vi "Entry_QueueOperations_FGV.vi"(8 "error in":errorcluster, 10 "Data":T1, 11 "Action":T3) -> (0 "error out":errorcluster, 1 "#elements in queue":i32, 2 "elements in queue":T1[](array[typedef]), 3 "queue ref":refnum<queue>)   [LabVIEW 2019]
uses:
  #typedef_Queue_enum.ctl
  #typedef_Data_Entry.ctl
  #typedef_EntryConsole_Action_enum.ctl
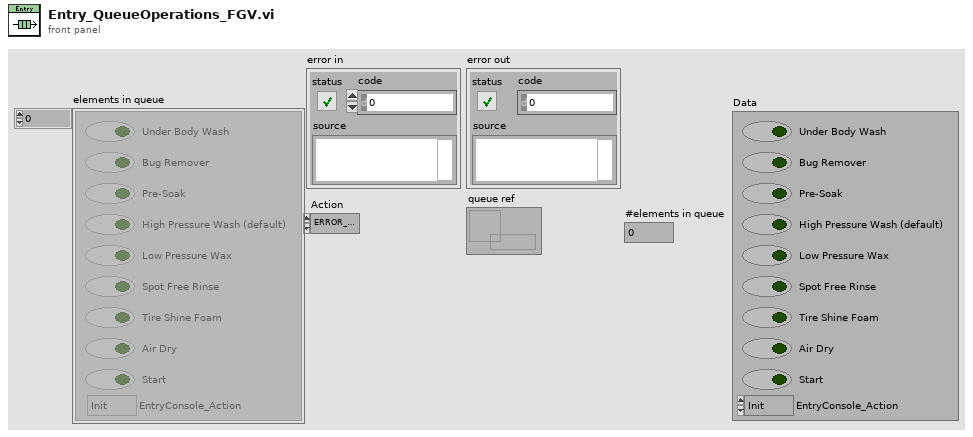
[diagram p1: front panel]
types:
  T1 = typedef "#typedef_Data_Entry.ctl" = cluster{"Under Body Wash":bool, "Bug Remover":bool, "Pre-Soak":bool, "High Pressure Wash (default)":bool, "Low Pressure Wax":bool, "Spot Free Rinse":bool, "Tire Shine Foam":bool, "Air Dry":bool, "Start":bool, "EntryConsole_Action":T2}
  T2 = typedef "#typedef_EntryConsole_Action_enum.ctl" = enum16{"Init", "ERROR_DEFAULT", "Idle", "Pending_Wash_Cycle", "Clear_Console", "Close", "Error_Handler", "Exit"}
  T3 = typedef "#typedef_Queue_enum.ctl" = enum16{"ERROR_default", "Obtain", "Enqueue", "GetStatus", "Flush", "Release"}
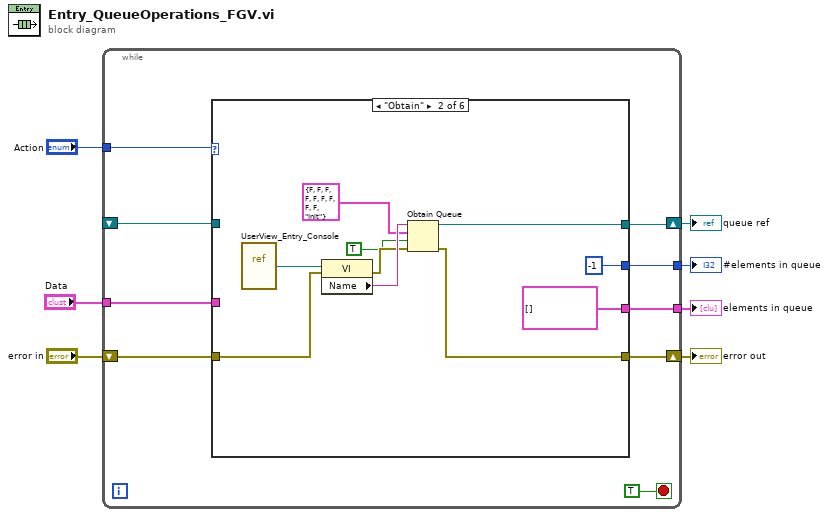
[diagram p0: block diagram]
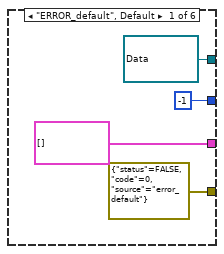
[diagram p2: hidden frame]
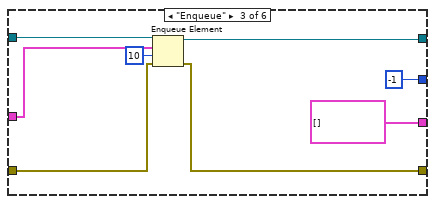
[diagram p3: hidden frame]
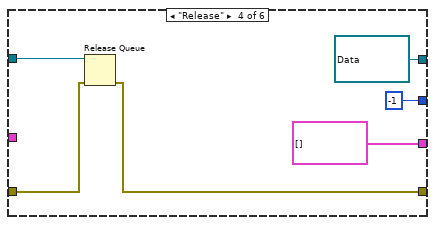
[diagram p4: hidden frame]
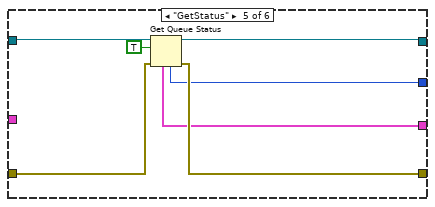
[diagram p5: hidden frame]
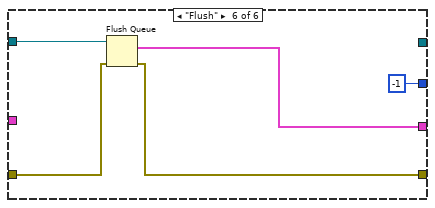
[diagram p6: hidden frame]
diagram:
  n1 = while {
    tunnel: "Action" -> [w15]
    tunnel: "Data" -> [w13]
    tunnel: [w10] -> w1
    shift-right: [w11] -> w3
    shift-left: _ -> [w9]
    shift-right: [w12] -> w5
    shift-left: "error in" -> [w14]
    tunnel: [w8] -> w2
    stop <- TRUE stop-if-true
    n2 = case shown="\"Obtain\"" w15 {
      tunnel: w14 -> [_ w30 w37 w43 w48 w55]
      tunnel: w13 -> [_ _ w33 _ _ _]
      tunnel: [errorcluster {"status"=FALSE, "code"=0, "source"="error_default"} ("error out") w27 w36 w42 w49 w54] -> w12
      tunnel: [refnum<queue> refnum ("queue out") w22 w35 refnum<queue> refnum ("queue out") w50 _] -> w11
      tunnel: [-1 ("# elements in queue") -1 ("#elements in queue") -1 ("#elements in queue") -1 ("# elements in queue") w47 -1 ("# elements in queue")] -> w10
      tunnel: w9 -> [_ _ w38 w44 w51 w56]
      tunnel: [T1[] [] ("Array") T1[] [] ("Array") T1[] [] ("Array") T1[] [] ("Array") w46 w52] -> w8
      frame "ERROR_default", Default {
      }
      frame "Obtain" {
        n3 = vi-ref "UserView_Entry_Console.vi"() -> (w24:refnum<vi>)
        n4 = property class="VI"(reference=w24, error in=w30) -> (error out=w28:errorcluster, "Name"=w29:string)  [unwired: 1 out]
        n5 = Obtain Queue(name (unnamed)=w29, element data type=T1 {"Under Body Wash"=FALSE, "Bug Remover"=FALSE, "Pre-Soak"=FALSE, "High Pressure Wash (default)"=FALSE, "Low Pressure Wax"=FALSE, "Spot Free Rinse"=FALSE, "Tire Shine Foam"=FALSE, "Air Dry"=FALSE, "Start"=FALSE, "EntryConsole_Action"=enum."Init"} ("Data"), create if not found? (T)=TRUE, error in (no error)=w28) -> (queue out=w22:refnum<queue>, error out=w27:errorcluster)  [unwired: 1 in, 1 out]
      }
      frame "Enqueue" {
        n6 = Enqueue Element(queue=w38, element=w33, timeout in ms (-1)=10, error in (no error)=w37) -> (queue out=w35:refnum<queue>, error out=w36:errorcluster)  [unwired: 1 out]
      }
      frame "Release" {
        n7 = Release Queue(queue=w44, error in (no error)=w43) -> (error out=w42:errorcluster)  [unwired: 1 in, 2 out]
      }
      frame "GetStatus" {
        n8 = Get Queue Status(queue=w51, return elements? (F)=TRUE, error in (no error)=w48) -> (queue out=w50:refnum<queue>, error out=w49:errorcluster, # elements in queue=w47:i32, elements=w46:T1[])  [unwired: 4 out]
      }
      frame "Flush" {
        n9 = Flush Queue(queue=w56, error in (no error)=w55) -> (remaining elements=w52:T1[], error out=w54:errorcluster)  [unwired: 1 out]
      }
    }
  }
  "error out" <- w5
  "#elements in queue" <- w1
  "elements in queue" <- w2
  "queue ref" <- w3
